vi "KYTION.vi"() -> ()   [LabVIEW 2018]
uses:
  <vilib>/Instr/_visa.llb/VISA Configure Serial Port (Instr).vi
panel:
  out "?":dbl(graph)
  out "Waveform Chart":dbl(graph)
  out "error out 3":errorcluster
  in  "VISA \nresource name":refnum<visa-resource-name>
  out "LOW HUMID":bool
  out "HIGH TEMP":bool
  in  "OPERATIONS":string(combo)
  out "WARNING":bool
  out "Humidity":dbl(slide) scale=0.0..100.0
  out "Temperature":dbl(slide) scale=0.0..50.0
  out "error out 2":errorcluster
  out "Read Buffer from KYTION's Serial Bus":string
  out "error out":errorcluster
  in  "XBee's\nCOM Port":refnum<visa-resource-name>
  in  "?":bool
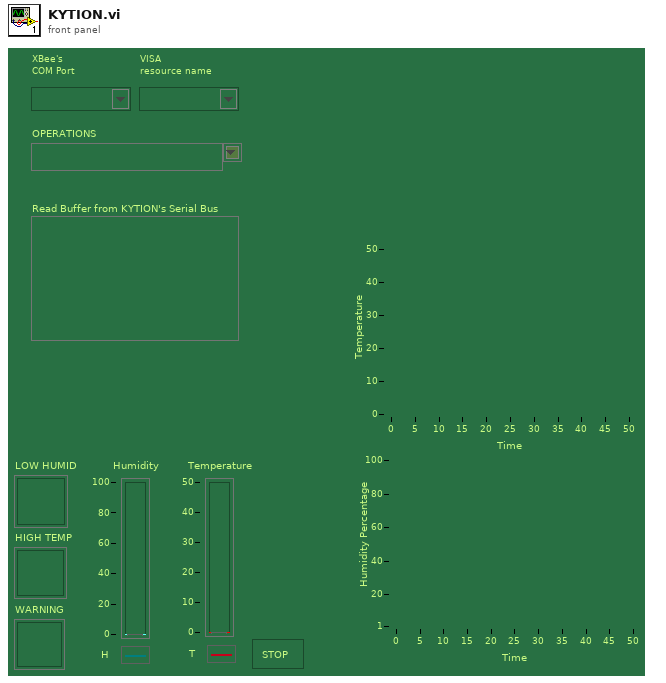
[diagram p1: front panel]
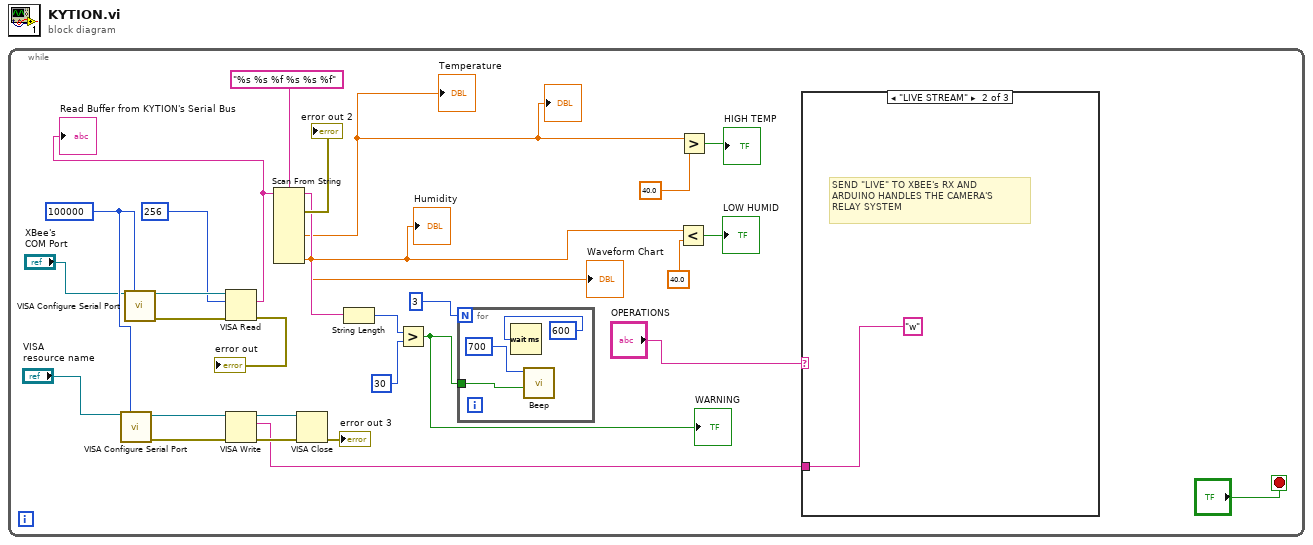
[diagram p0: block diagram]
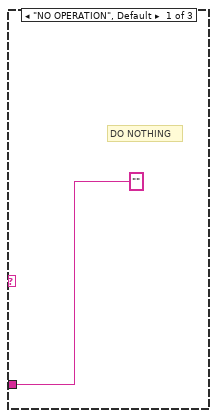
[diagram p2: hidden frame]
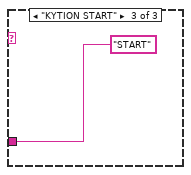
[diagram p3: hidden frame]
diagram:
  n1 = while {
    stop <- "?" stop-if-true
    w16 = u32 100000 ("timeout (10sec)")
    n2 = call-poly "VISA Configure Serial Port"("VISA resource name"="VISA \nresource name", "timeout (10sec)"=w16) -> ("VISA resource name out"=w15:refnum<visa-resource-name>, "error out"=w13:errorcluster)  [unwired: 12 in]
    n3 = call-poly "VISA Configure Serial Port"("VISA resource name"="XBee's\nCOM Port", "timeout (10sec)"=w16) -> ("VISA resource name out"=w28:refnum<visa-resource-name>, "error out"=w27:errorcluster)  [unwired: 12 in]
    n4 = VISA Read(VISA resource name=w28, byte count=u32 256, error in (no error)=w27) -> (read buffer=w24:string, error out=→"error out":errorcluster)  [unwired: 2 out]
    "Read Buffer from KYTION's Serial Bus" <- w24
    n5 = Scan From String(format string="%s %s %f %s %s %f", input string=w24) -> (remaining string=w21:string, error out=→"error out 2":errorcluster, output 3=w1:dbl, output 6=w2:dbl)  [unwired: 12 in, 1 out]
    "Temperature" <- w1
    "Humidity" <- w2
    "Waveform Chart" <- w2
    "?" <- w1
    n6 = String Length(string=w21) -> (length=w20:i32)
    n7 = Greater?(x=w20, y=30) -> (0:w17:bool)
    "WARNING" <- w17
    n8 = for {
      N: 3 -> [_]
      tunnel: w17 -> [w34]
      n9 = Wait (ms)(milliseconds to wait=u32 600 ("millisecond timer value")) -> ()  [unwired: 1 out]
      n10 = call <vilib>:"Beep.vi"("use system alert? (T)"=w34, "frequency (Hz)"=u32 700) -> ()  [unwired: 10 in]
    }
    n11 = Less?(x=w2, y=40.0) -> (x < y?=→"LOW HUMID":bool)
    n12 = Greater?(x=w1, y=40.0) -> (0:→"HIGH TEMP":bool)
    n13 = case shown="\"LIVE STREAM\"" "OPERATIONS" {
      tunnel: ["" ("write buffer") "w" ("write buffer") "START" ("write buffer")] -> w9
      frame "NO OPERATION", Default {
        # "DO NOTHING"
      }
      frame "LIVE STREAM" {
        # "SEND \"LIVE\" TO XBEE's RX AND\nARDUINO HANDLES THE CAMERA'S\nRELAY SYSTEM"
      }
      frame "KYTION START" {
      }
    }
    n14 = VISA Write(VISA resource name=w15, write buffer=w9, error in (no error)=w13) -> (VISA resource name out=w11:refnum<visa-resource-name>, error out=w12:errorcluster)  [unwired: 1 out]
    n15 = VISA Close(VISA resource name=w11, error in (no error)=w12) -> (error out=→"error out 3":errorcluster)
  }
